vi "RSZVB Get Default Configuration State.vi"(8 "error in (no error)":errorcluster {"code" format="%.0x"}, 11 "VISA session":refnum<visa-resource-name>) -> (0 "error out":errorcluster {"code" format="%.0x"}, 1 "Default Settings":bool, 3 "dup VISA session":refnum<visa-resource-name>)   [LabVIEW 2011]
doc: "This VI returns the default configuration state\n\nRemote-control command(s):\nROUTe<Ch>:CFILe?"
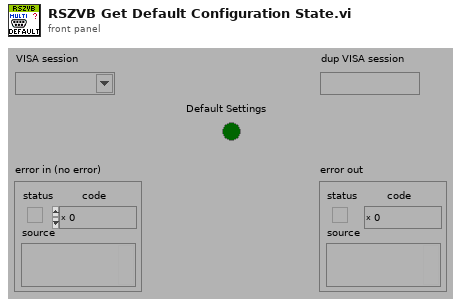
[diagram p1: front panel]
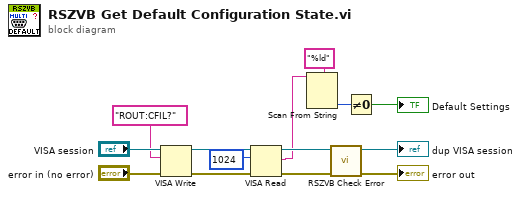
[diagram p0: block diagram]
diagram:
  n1 = VISA Write(VISA resource name="VISA session", write buffer="ROUT:CFIL?", error in (no error)="error in (no error)") -> (VISA resource name out=w11:refnum<visa-resource-name>, error out=w10:errorcluster)  [unwired: 1 out]
  n2 = VISA Read(VISA resource name=w11, byte count=u32 1024 ("byte count (0)"), error in (no error)=w10) -> (VISA resource name out=w5:refnum<visa-resource-name>, read buffer=w1:string, error out=w8:errorcluster)  [unwired: 1 out]
  n3 = Scan From String(format string="%ld", input string=w1) -> (output 1=w3:i32)  [unwired: 3 in, 3 out]
  n4 = call "RSZVB Check Error.vi"("error in (no error)"=w8, "VISA session"=w5) -> ("error out"=→"error out":errorcluster, "dup VISA session"=→"dup VISA session":refnum<visa-resource-name>)  [unwired: 8 in]
  n5 = Not Equal To 0?(x=w3) -> (x != 0?=→"Default Settings":bool)
